vi "Acquisition.vi"() -> ()   [LabVIEW 2009]
panel:
  out "Iterations":i32(slide) scale=0.0..2.0
  out "Integration":i32(slide) scale=0.0..100.0
  in  "Iterations":i32
  in  "Dark Duration":i32
  in  "Fringes Duration":i32
  in  "Ratio Duration":i32
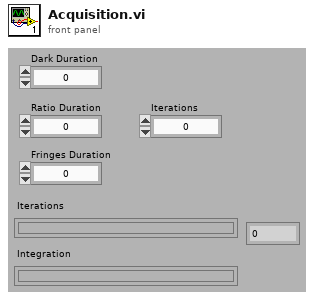
[diagram p1: front panel]
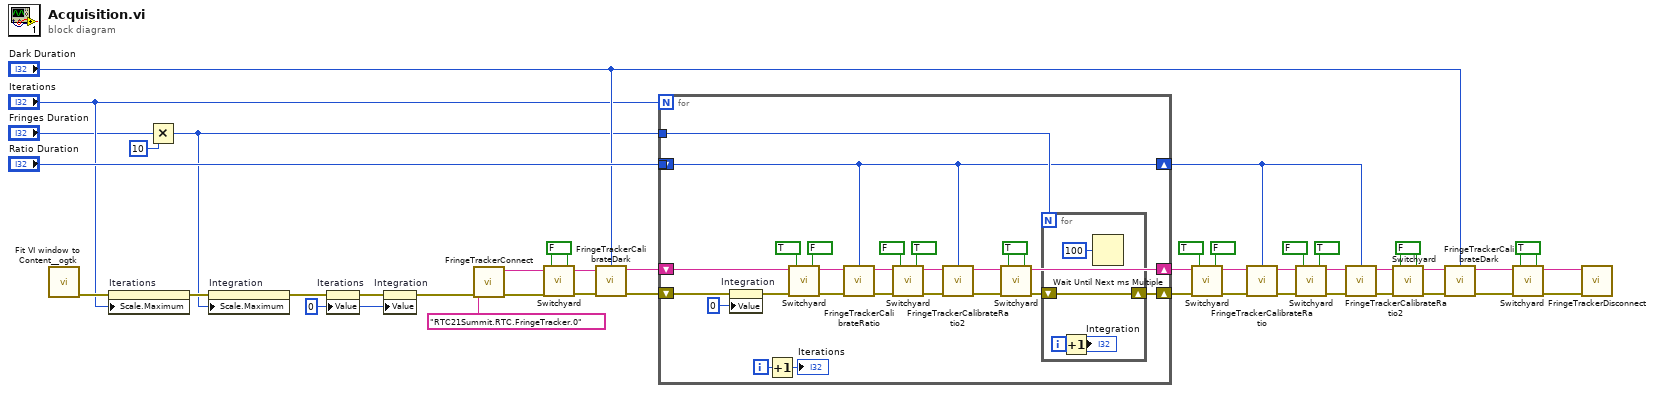
[diagram p0: block diagram]
diagram:
  w19 = 0 ("Iterations")
  w31 = TRUE ("K1")
  w33 = FALSE ("K1")
  w35 = FALSE ("K1")
  n1 = call <userlib>:"Fit VI window to Content__ogtk.vi"() -> ("error out"=w24:errorcluster)  [unwired: 3 in, 4 out]
  n2 = property on="Iterations" class="Slide (strict)"(error in=w24, "Scale.Maximum"="Iterations") -> (error out=w22:errorcluster)  [unwired: 1 in, 1 out]
  n3 = Multiply(x="Fringes Duration", y=10) -> (x*y=w15:i32)
  n4 = property on="Integration" class="Slide (strict)"(error in=w22, "Scale.Maximum"=w15) -> (error out=w21:errorcluster)  [unwired: 1 in, 1 out]
  n5 = property on="Iterations" class="Slide (strict)"(error in=w21, "Value"=w19) -> (error out=w20:errorcluster)  [unwired: 1 in, 1 out]
  n6 = property on="Integration" class="Slide (strict)"(error in=w20, "Value"=w19) -> (error out=w18:errorcluster)  [unwired: 1 in, 1 out]
  n7 = call "FringeTrackerConnect.vi"("FringeTracker Name"="RTC21Summit.RTC.FringeTracker.0", "error in (no error)"=w18) -> ("FringeTracker Name out"=w28:string, "error out"=w29:errorcluster)  [unwired: 6 out]
  n8 = call "Switchyard.vi"("K2"=w35, "K1"=w35, "error in (no error)"=w29) -> ("error out"=w36:errorcluster)  [unwired: 4 out]
  n9 = call "FringeTrackerCalibrateDark.vi"("Seconds"="Dark Duration", "FringeTracker Name"=w28, "error in (no error)"=w36) -> ("FringeTracker Name out"=w34:string, "error out"=w37:errorcluster)  [unwired: 5 out]
  n10 = for {
    N: "Iterations" -> [_]
    tunnel: "Ratio Duration" -> [w39]
    tunnel: w15 -> [w40]
    shift-right: [w46] -> w6
    shift-left: w37 -> [w43]
    shift-right: [w47] -> w5
    shift-left: w34 -> [w58]
    shift-right: [w39] -> w1
    shift-left: _ -> [_]
    i -> [w45]
    w49 = TRUE ("K1")
    n11 = property on="Integration" class="Slide (strict)"(error in=w43, "Value"=0 ("Integration")) -> (error out=w42:errorcluster)  [unwired: 1 in, 1 out]
    n12 = Increment(x=w45) -> (x+1=→"Iterations":i32)
    n13 = call "Switchyard.vi"("K2"=FALSE ("K1"), "K1"=TRUE, "error in (no error)"=w42) -> ("error out"=w59:errorcluster)  [unwired: 4 out]
    n14 = call "FringeTrackerCalibrateRatio.vi"("Seconds"=w39, "FringeTracker Name"=w58, "error in (no error)"=w59) -> ("FringeTracker Name out"=w57:string, "error out"=w51:errorcluster)  [unwired: 5 out]
    n15 = call "Switchyard.vi"("K2"=TRUE ("K1"), "K1"=FALSE, "error in (no error)"=w51) -> ("error out"=w52:errorcluster)  [unwired: 4 out]
    n16 = call "FringeTrackerCalibrateRatio2.vi"("Seconds"=w39, "FringeTracker Name"=w57, "error in (no error)"=w52) -> ("FringeTracker Name out"=w47:string, "error out"=w50:errorcluster)  [unwired: 5 out]
    n17 = call "Switchyard.vi"("K2"=w49, "K1"=w49, "error in (no error)"=w50) -> ("error out"=w48:errorcluster)  [unwired: 4 out]
    n18 = for {
      N: w40 -> [_]
      shift-right: [w63] -> w46
      shift-left: w48 -> [w63]
      i -> [w61]
      n19 = Increment(x=w61) -> (x+1=→"Integration":i32)
      n20 = Wait Until Next ms Multiple(millisecond multiple=u32 100) -> ()  [unwired: 1 out]
    }
  }
  n21 = call "Switchyard.vi"("K2"=FALSE ("K1"), "K1"=TRUE, "error in (no error)"=w6) -> ("error out"=w7:errorcluster)  [unwired: 4 out]
  n22 = call "FringeTrackerCalibrateRatio.vi"("Seconds"=w1, "FringeTracker Name"=w5, "error in (no error)"=w7) -> ("FringeTracker Name out"=w8:string, "error out"=w14:errorcluster)  [unwired: 5 out]
  n23 = call "Switchyard.vi"("K2"=TRUE ("K1"), "K1"=FALSE, "error in (no error)"=w14) -> ("error out"=w13:errorcluster)  [unwired: 4 out]
  n24 = call "FringeTrackerCalibrateRatio2.vi"("Seconds"=w1, "FringeTracker Name"=w8, "error in (no error)"=w13) -> ("FringeTracker Name out"=w4:string, "error out"=w3:errorcluster)  [unwired: 5 out]
  n25 = call "Switchyard.vi"("K2"=w33, "K1"=w33, "error in (no error)"=w3) -> ("error out"=w2:errorcluster)  [unwired: 4 out]
  n26 = call "FringeTrackerCalibrateDark.vi"("Seconds"="Dark Duration", "FringeTracker Name"=w4, "error in (no error)"=w2) -> ("FringeTracker Name out"=w26:string, "error out"=w30:errorcluster)  [unwired: 5 out]
  n27 = call "Switchyard.vi"("K2"=w31, "K1"=w31, "error in (no error)"=w30) -> ("error out"=w25:errorcluster)  [unwired: 4 out]
  n28 = call "FringeTrackerDisconnect.vi"("FringeTracker Name"=w26, "error in (no error)"=w25) -> ()  [unwired: 8 out]
